vi "Get Number DDG External Outputs.vi"(11 "puiCount":u32) -> (2 "function return":u32, 3 "puiCount out":u32)   [LabVIEW 2018, in "Copy of Andor SDK.lvlib"]
doc: "EXPNETTYPE unsigned int WINAPI GetNumberDDGExternalOutputs(at_u32 * puiCount);"
uses:
  Copy of Andor SDK.lvlib
  <userlib>/Andor SDK/ATMCD32D.dll
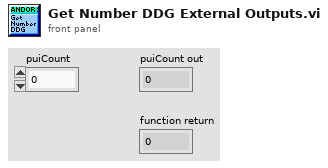
[diagram p1: front panel]
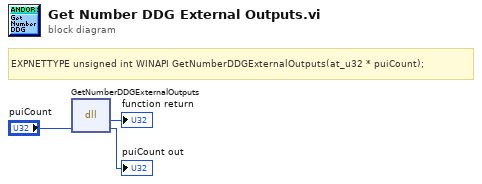
[diagram p0: block diagram]
diagram:
  # "EXPNETTYPE unsigned int WINAPI GetNumberDDGExternalOutputs(at_u32 * puiCount);"
  n1 = dll-call lib="C:/Program Files (x86)/National Instruments/LabVIEW 2018/user.lib/Andor SDK/ATMCD32D.*" fn="GetNumberDDGExternalOutputs"("puiCount"="puiCount") -> (→"function return":u32, "puiCount"=→"puiCount out":u32)  [unwired: 3 in, 2 out]
